vi "Pswd creator.vi"() -> ()   [LabVIEW 2012]
uses:
  SubVIs/typedef/User Accounts.ctl
  SubVIs/typedef/User_Data_Cluster.ctl
panel:
  out "Array":T1[](array[typedef])
  out "UD array":string[](array[string])
  out "User-data cluster":T1
  in  "?":T3={"Usuario"="None", "Password"="1234aAaA!", "Account type"=enum."None"}
  in  "?":bool
  out "CypheredText":string
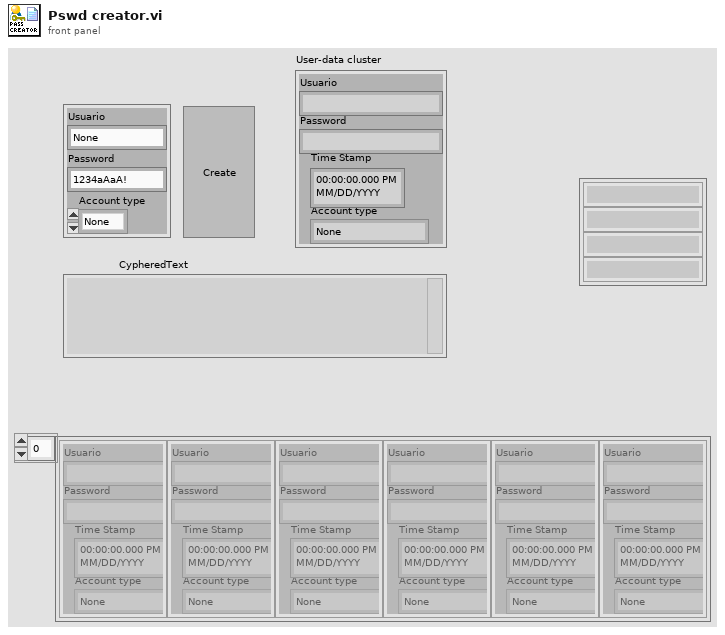
[diagram p1: front panel]
types:
  T1 = typedef "User_Data_Cluster.ctl" = cluster{"Usuario":string, "Password":string, "Account type":T2, "Time Stamp":timestamp}
  T2 = typedef "User Accounts.ctl" = enum16{"None", "User", "Admin"}
  T3 = cluster{"Usuario":string, "Password":string, "Account type":T2}
  T4 = enum16{"open", "replace", "create", "open or create", "replace or create", "replace or create with confirmation"}
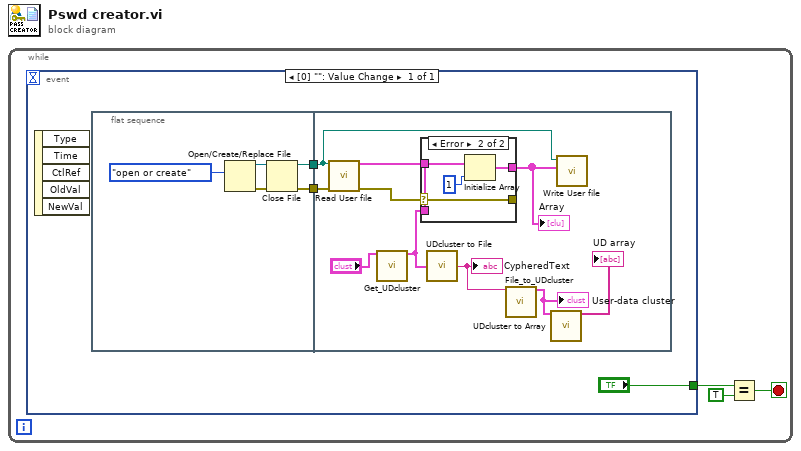
[diagram p0: block diagram]
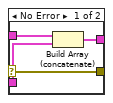
[diagram p2: hidden frame]
diagram:
  n1 = while {
    stop <- w3 stop-if-true
    n2 = event shown="[0] \"\": Value Change" {
      selector: _ -> [_]
      dyn-events: _ -> [_]
      timeout: _ -> [_]
      tunnel: ["?"] -> w1
      event Value Change {
        n3 = event-data() -> ()  [unwired: 1 in, 5 out]
        n4 = flat-sequence {
          tunnel: [w8] -> w5
          tunnel: [w7] -> w4
          tunnel: w5 -> [w20]
          tunnel: w4 -> [w19]
          frame #0 {
            n5 = Open/Create/Replace File(operation (0:open)=T4."open or create") -> (refnum out=w11:refnum<file>, error out=w9:errorcluster)  [unwired: 5 in, 1 out]
            n6 = Close File(refnum=w11, error in=w9) -> (path=w8:path, error out=w7:errorcluster)
          }
          frame #1 {
            n7 = call "Read User file.vi"("file path (use dialog)"=w20, "error in"=w19) -> ("Array"=w21:T1[], "error out"=w18:errorcluster)  [unwired: 12 in]
            n8 = call "Get_UDcluster.vi"("Cluster"="?") -> ("User-data cluster out"=w17:T1)  [unwired: 13 in, 1 out]
            n9 = case shown="Error" w18 {
              selector: w18 -> [w22 w26]
              tunnel: w21 -> [w25 _]
              tunnel: [w24 w27] -> w12
              tunnel: w17 -> [w23 w28]
              tunnel: [w22 w26] -> _
              frame No Error {
                n10 = Build Array (concatenate)(w25, w23) -> (w24:T1[])
              }
              frame Error {
                n11 = Initialize Array(w28, 1 ("dimension size")) -> (w27:T1[])
              }
            }
            "Array" <- w12
            n12 = call "UDcluster to File.vi"("User-data cluster"=w17) -> ("CypheredText"=w15:string)
            "CypheredText" <- w15
            n13 = call "File_to_UDcluster.vi"("Cyphered text"=w15) -> ("User-data cluster"=w14:T1)  [unwired: 13 in, 1 out]
            "User-data cluster" <- w14
            n14 = call "UDcluster to Array.vi"("User-data cluster"=w14) -> ("UD array"=→"UD array":string[])  [unwired: 13 in, 1 out]
            n15 = call "Write User file.vi"("Array"=w12, "file path (use dialog)"=w20) -> ()  [unwired: 8 in, 2 out]
          }
        }
      }
    }
    n16 = Equal?(x=w1, y=TRUE) -> (x = y?=w3:bool)
  }
